vi "test2.vi"() -> ()   [LabVIEW 2014]
uses:
  picohrdl.dll
panel:
  out "P5":dbl[](graph)
  out "P4":dbl[](graph)
  out "P3":dbl[](graph)
  out "P2":dbl[](graph)
  out "P1":dbl[](graph)
  in  "Voltage range":i32[](array[numeric])=[6, 0, 0, 0, 0, 0, 0, 0, 3, 0, 0, 0, 0, 0, 0, 0] min=0 max=6 step=1
  in  "Single ended\n(1- single)\n(0 - difer)":i32[](array[numeric])=[0, 1, 1, 1, 1, 1, 1, 1, 1, 1, 1, 1, 1, 1, 1, 1] min=0 max=1 step=1
  in  "Ch nr":bool[](array[boolean])=[TRUE, FALSE, FALSE, FALSE, TRUE, FALSE, TRUE, FALSE, TRUE, FALSE, TRUE, FALSE, FALSE, FALSE, FALSE, FALSE]
  in  "conversionTime":i16(ring)=3 items=["60 ms", "100 ms", "180 ms", "340 ms", "660 ms"]
  in  "Mains Frequency":i16(ring) items=["50 Hz", "60 Hz"]
  out "Waveform Graph 3":dynamicdata(graph)
  in  "sampleInterval_ms":i32=2500
  in  "stop":bool
  # "1       2       3      4       5        6       7       8       9      10     11      12     13    14       15     16"
  # "0 -+2500mV\n1 -+1250mV\n2 -+625mV\n3 -+313mV\n4 -+156mV\n5 -+78mv\n6 -+39mV"
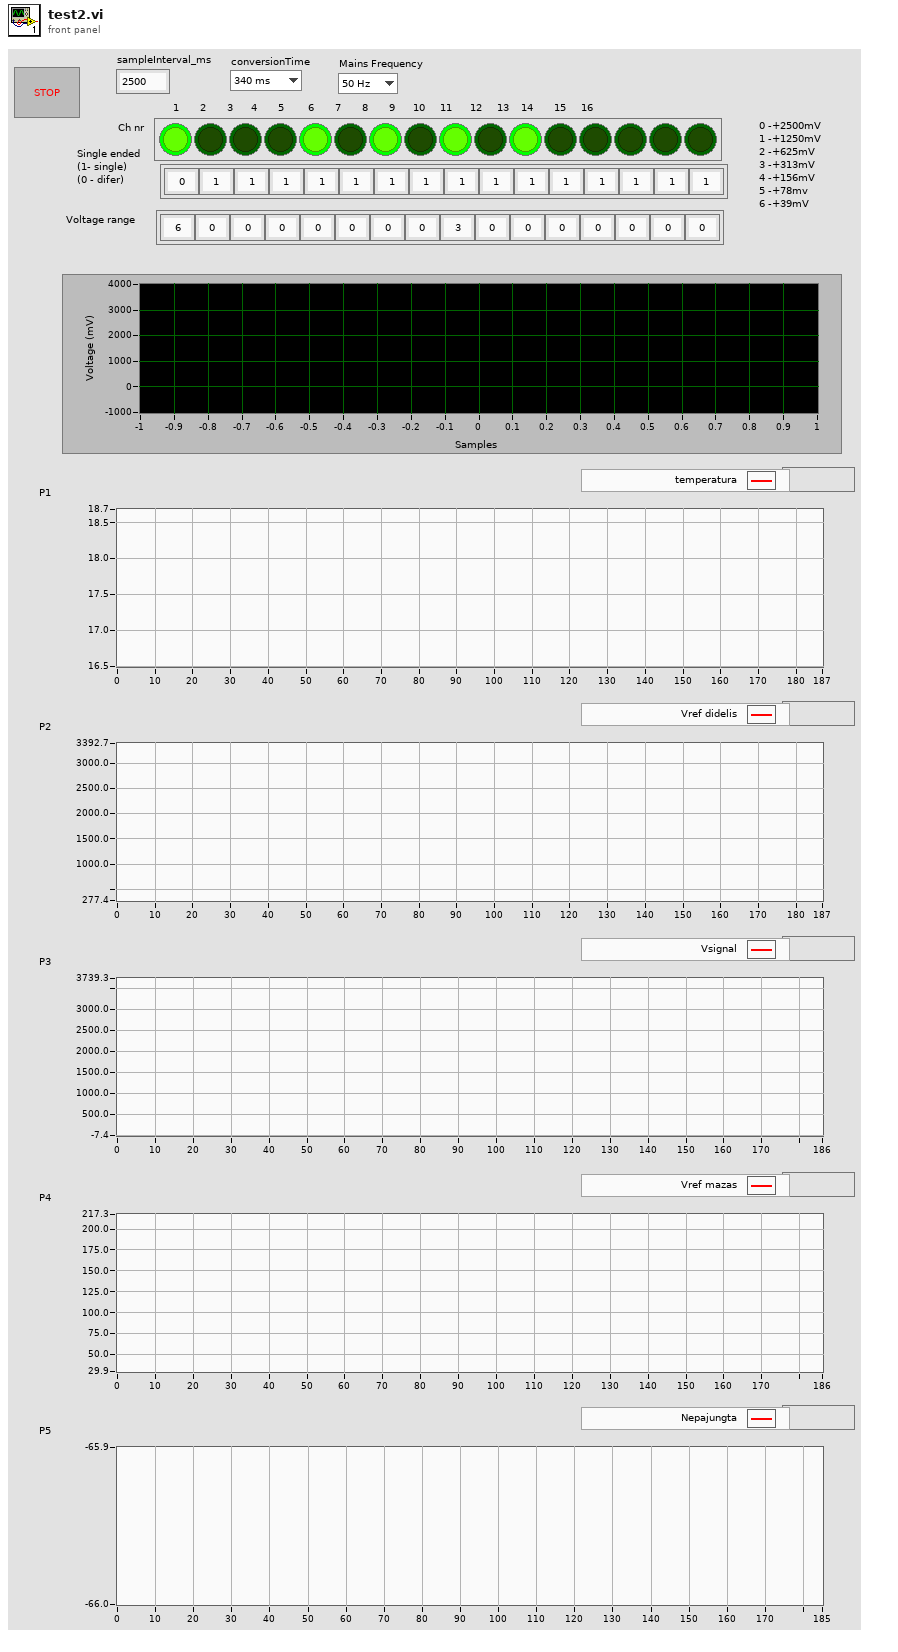
[diagram p1: front panel]
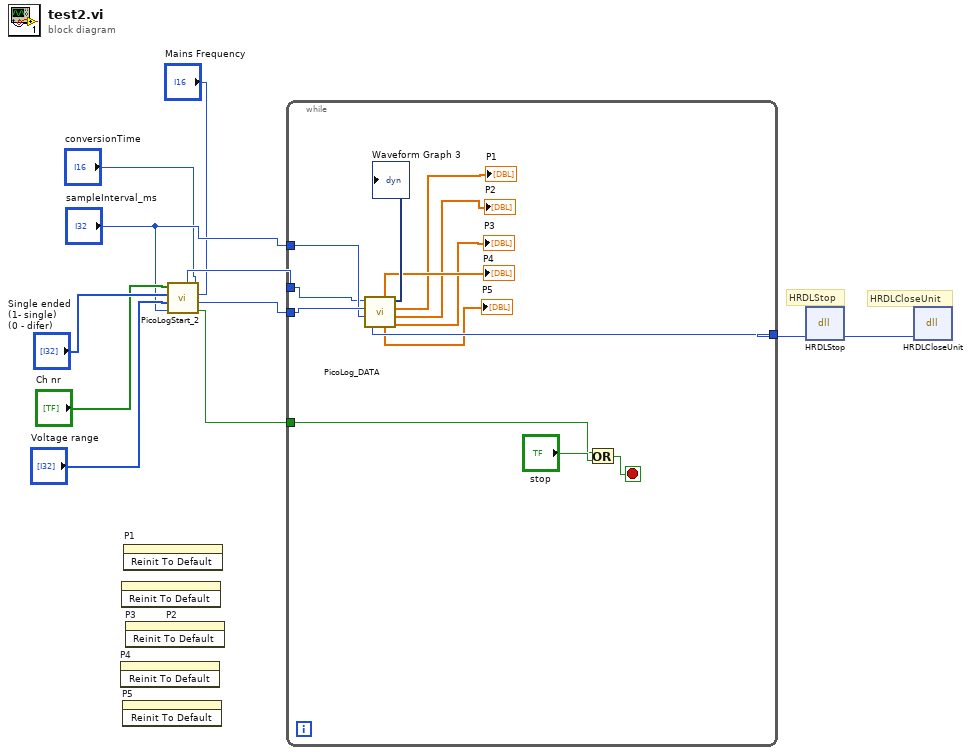
[diagram p0: block diagram]
diagram:
  # "HRDLStop"
  # "HRDLCloseUnit"
  n1 = invoke on="P4" class="WFChart (strict)" method="Reinit To Default"() -> ()  [unwired: 3 in, 3 out]
  n2 = invoke on="P2" class="WFChart (strict)" method="Reinit To Default"() -> ()  [unwired: 3 in, 3 out]
  n3 = invoke on="P5" class="WFChart (strict)" method="Reinit To Default"() -> ()  [unwired: 3 in, 3 out]
  n4 = invoke on="P1" class="WFChart (strict)" method="Reinit To Default"() -> ()  [unwired: 3 in, 3 out]
  n5 = invoke on="P3" class="WFChart (strict)" method="Reinit To Default"() -> ()  [unwired: 3 in, 3 out]
  n6 = call "PicoLogStart_2.vi"("Ch nr"="Ch nr", "Single ended\n(0- single)\n(1 - difer)"="Single ended\n(1- single)\n(0 - difer)", "Voltage range"="Voltage range", "sampleInterval_ms"="sampleInterval_ms", "conversionTime"="conversionTime", "Mains Frequency"="Mains Frequency") -> ("noOfChannels"=w8:i16, "handle"=w9:i16, "STOP"=w1:bool)
  n7 = while {
    tunnel: w9 -> [w24]
    tunnel: "sampleInterval_ms" -> [w23]
    tunnel: w1 -> [w19]
    tunnel: [w18] -> w10
    tunnel: w8 -> [w17]
    stop <- w21 stop-if-true
    n8 = call "PicoLog_DATA.vi"("noOfChannels"=w17, "handle"=w24, "sampleInterval_ms"=w23) -> ("handle"=w18:i16, "P4"=→"P4":dbl[], "P5"=→"P5":dbl[], "Waveform Graph 3"=→"Waveform Graph 3":dynamicdata, "P1"=→"P1":dbl[], "P2"=→"P2":dbl[], "P3"=→"P3":dbl[])
    n9 = Or(x=w19, y="stop") -> (x .or. y?=w21:bool)
  }
  n10 = dll-call lib="picohrdl.dll" fn="HRDLStop"("handle"=w10) -> ("handle"=w11:i16)  [unwired: 4 in, 2 out]
  n11 = dll-call lib="PicoHRDL.dll" fn="HRDLCloseUnit"("handle"=w11) -> ()  [unwired: 5 in, 2 out]
